vi "GamePlayfield_LineClear.vi"(2 "Player":u8) -> (16 "LinesCleared":u8)   [LabVIEW 2018]
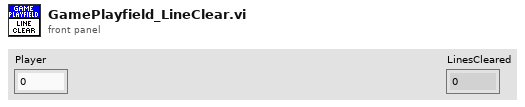
[diagram p1: front panel]
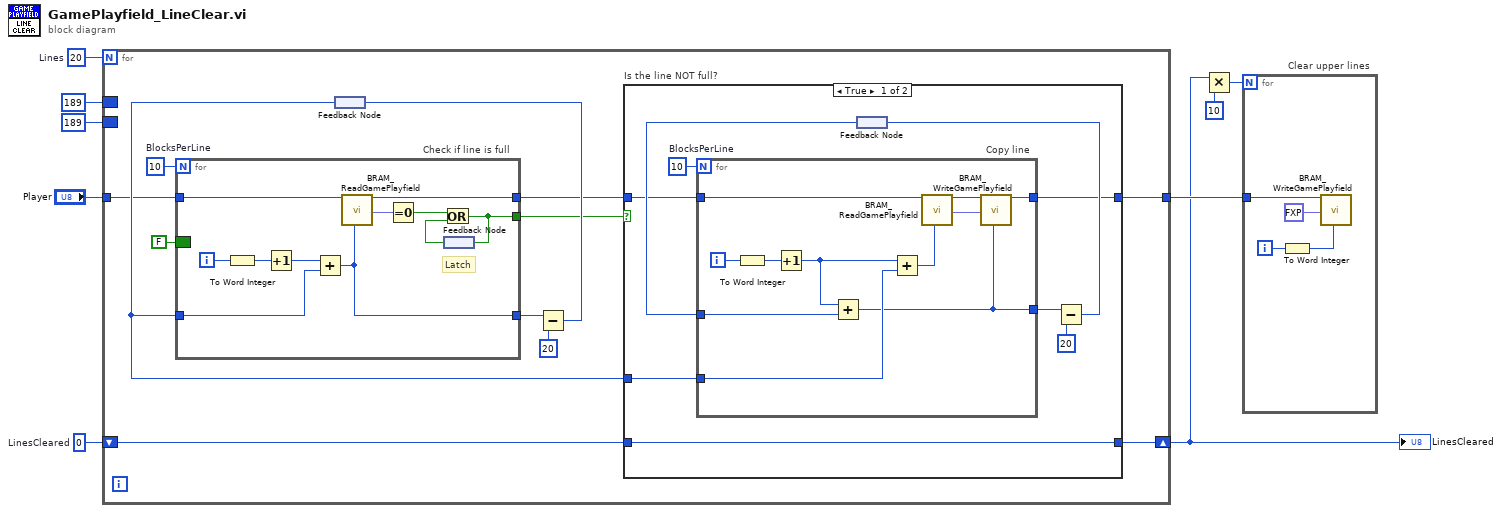
[diagram p0: block diagram]
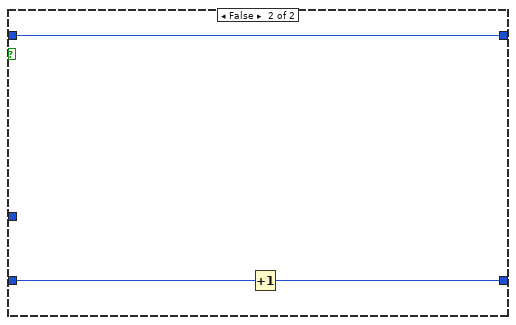
[diagram p2: hidden frame]
diagram:
  w8 = u8 0  # LinesCleared
  w9 = 20  # Lines
  n1 = for {
    N: w9 -> [_]
    shift-right: [w19] -> w1
    shift-left: w8 -> [w20]
    border: i16 189 -> [_]
    border: i16 189 -> [_]
    tunnel: "Player" -> [w12]
    tunnel: [w10] -> w4
    w21 = 10  # BlocksPerLine
    n2 = feedback #1() -> (w13:i16)
    n3 = for "Check if line is full" {
      N: w21 -> [_]
      tunnel: [w28] -> w17
      border: FALSE -> [_]
      tunnel: w13 -> [w31]
      tunnel: [w26] -> w14
      tunnel: w12 -> [w27]
      tunnel: [w22] -> w11
      i -> [w32]
      # "Latch"
      n4 = To Word Integer(number=w32) -> (16bit integer=w30:i16)
      n5 = Increment(x=w30) -> (x+1=w29:i16)
      n6 = Add(x=w29, y=w31) -> (x+y=w26:i16)
      n7 = call "BRAM_ReadGamePlayfield.vi"("Player IN"=w27, "Address"=w26) -> ("Player OUT"=w22:u8, "Data"=w25:fxp<+,3,3>)  [unwired: 16 in]
      n8 = Equal To 0?(x=w25) -> (x = 0?=w23:bool)
      n9 = feedback #2() -> (w24:bool)
      n10 = Or(x=w23, y=w24) -> (x .or. y?=w28:bool)
      n11 = feedback-in #2(w28) -> ()
    }
    n12 = Subtract(x=w14, y=i16 20) -> (x-y=w18:i16)
    n13 = feedback-in #1(w18) -> ()
    n14 = case "Is the line NOT full?" shown="True" w17 {
      tunnel: w20 -> [w40 w55]
      tunnel: [w40 w54] -> w19
      tunnel: w13 -> [w37 _]
      tunnel: w11 -> [w34 w53]
      tunnel: [w33 w53] -> w10
      frame True {
        w41 = 10  # BlocksPerLine
        n15 = feedback #3() -> (w36:i16)
        n16 = for "Copy line" {
          N: w41 -> [_]
          tunnel: w37 -> [w49]
          tunnel: [w45] -> w38
          tunnel: w36 -> [w48]
          tunnel: w34 -> [w47]
          tunnel: [w42] -> w33
          i -> [w52]
          n17 = To Word Integer(number=w52) -> (16bit integer=w51:i16)
          n18 = Increment(x=w51) -> (x+1=w50:i16)
          n19 = Add(x=w50, y=w48) -> (x+y=w45:i16)
          n20 = Add(x=w50, y=w49) -> (x+y=w46:i16)
          n21 = call "BRAM_ReadGamePlayfield.vi"("Player IN"=w47, "Address"=w46) -> ("Player OUT"=w43:u8, "Data"=w44:fxp<+,3,3>)  [unwired: 16 in]
          n22 = call "BRAM_WriteGamePlayfield.vi"("Player IN"=w43, "Data"=w44, "Address"=w45) -> ("Player OUT"=w42:u8)  [unwired: 16 in]
        }
        n23 = Subtract(x=w38, y=i16 20) -> (x-y=w35:i16)
        n24 = feedback-in #3(w35) -> ()
      }
      frame False {
        n25 = Increment(x=w55) -> (x+1=w54:u8)
      }
    }
  }
  "LinesCleared" <- w1
  n26 = Multiply(x=w1, y=u8 10) -> (x*y=w3:u8)
  n27 = for "Clear upper lines" {
    N: w3 -> [_]
    tunnel: w4 -> [w57]
    i -> [w59]
    n28 = To Word Integer(number=w59) -> (16bit integer=w58:i16)
    n29 = call "BRAM_WriteGamePlayfield.vi"("Player IN"=w57, "Data"=fxp<+,3,3> 0.0, "Address"=w58) -> ()  [unwired: 16 in, 1 out]
  }
